vi "Percent-Encode String.vi"(10 "String":string) -> (2 "Pct-Encoded String":string)   [LabVIEW 2013, in "openURI.lvlib"]
uses:
  openURI.lvlib
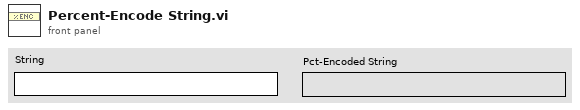
[diagram p1: front panel]
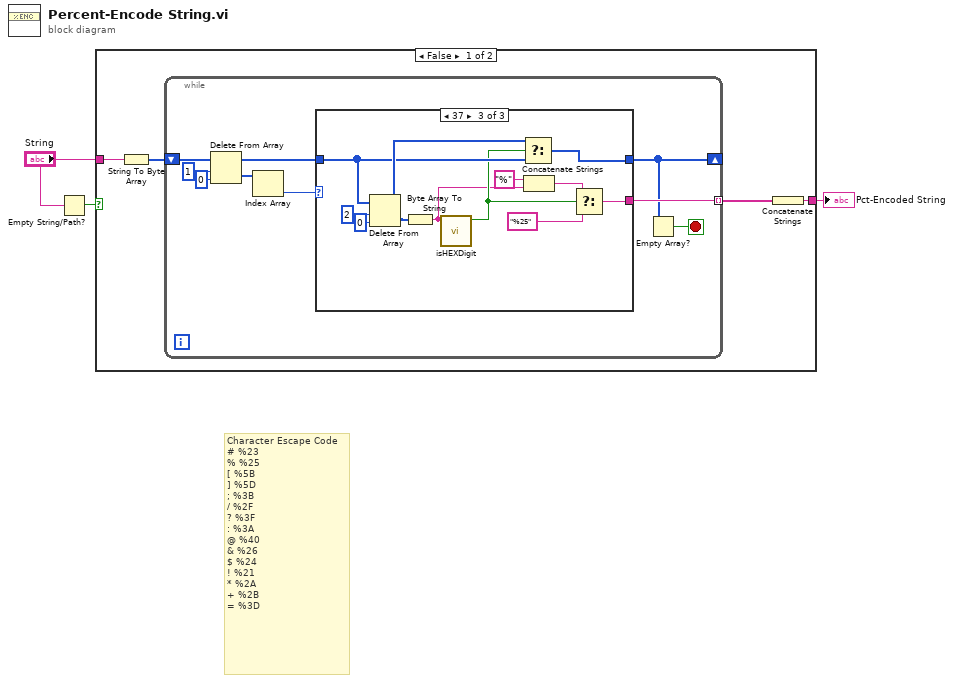
[diagram p0: block diagram]
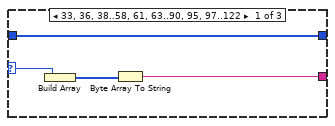
[diagram p2: hidden frame]
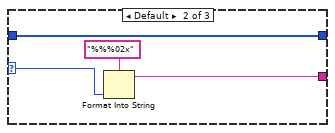
[diagram p3: hidden frame]
diagram:
  # "Character\tEscape Code\n#\t%23\n%\t%25\n[\t%5B\n]\t%5D\n;\t%3B\n/\t%2F\n?\t%3F\n:\t%3A\n@\t%40\n&\t%26\n$\t%24\n!\t%21\n*\t%2A\n+\t%2B\n=\t%3D"
  n1 = Empty String/Path?(string/path="String") -> (empty?=w2:bool)
  n2 = case shown="False" w2 {
    tunnel: "String" -> [w5 _]
    tunnel: [w4 _] -> w3
    frame False {
      n3 = String To Byte Array(string=w5) -> (unsigned byte array=w7:u8[])
      n4 = while {
        tunnel: [w16] -> w6 mode=indexing
        shift-right: [w9] -> _
        shift-left: w7 -> [w15]
        stop <- w8 stop-if-true
        n5 = Delete From Array(array=w15, length=1, index=0) -> (deleted portion=w12:u8[], array with subset deleted=w10:u8[])
        n6 = Index Array(array=w12) -> (element=w11:u8)  [unwired: 1 in]
        n7 = case shown="37" w11 {
          selector: w11 -> [w20 w24 _]
          tunnel: [w18 w22 w29] -> w16
          tunnel: w10 -> [w17 w21 w32]
          tunnel: [w17 w21 w31] -> w9
          frame 33, 36, 38..58, 61, 63..90, 95, 97..122 {
            n8 = Build Array(w20) -> (w19:u8[])
            n9 = Byte Array To String(unsigned byte array=w19) -> (string=w18:string)
          }
          frame Default {
            n10 = Format Into String(format string="%%%02x", w24) -> (resulting string=w22:string)  [unwired: 2 in, 1 out]
          }
          frame 37 {
            n11 = Delete From Array(array=w32, length=2, index=0) -> (deleted portion=w34:u8[], array with subset deleted=w33:u8[])
            n12 = Byte Array To String(unsigned byte array=w34) -> (string=w27:string)
            n13 = call "isHEXDigit.vi"("characters"=w27) -> ("HEX Digits"=w30:bool)  [unwired: 10 in]
            n14 = Select(t=w33, s=w30, f=w32) -> (s? t:f=w31:u8[])
            n15 = Concatenate Strings("%" ("string"), w27) -> (w26:string)
            n16 = Select(t=w26, s=w30, f="%25" ("string")) -> (s? t:f=w29:string)
          }
        }
        n17 = Empty Array?(array=w9) -> (empty?=w8:bool)
      }
      n18 = Concatenate Strings(w6) -> (w4:string)
    }
    frame True {
    }
  }
  "Pct-Encoded String" <- w3
